vi "KM_String Array Select.vi"(10 "Selector array":bool[](array[boolean]), 11 "Full array":string[](array[string])) -> (3 "Array":string[](array[string]))   [LabVIEW 2015]
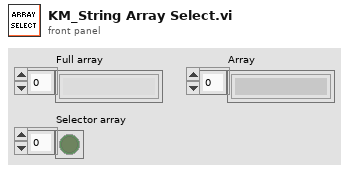
[diagram p1: front panel]
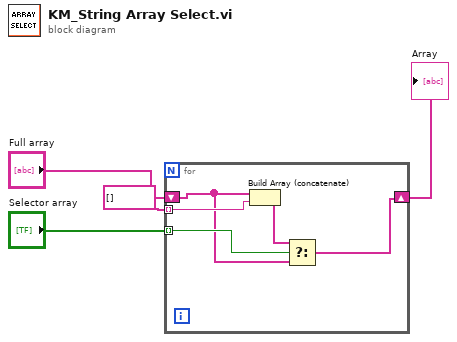
[diagram p0: block diagram]
diagram:
  n1 = for {
    tunnel: "Full array" -> [w8] mode=indexing
    tunnel: "Selector array" -> [w9] mode=indexing
    shift-right: [w5] -> w2
    shift-left: string[] [] -> [w6]
    n2 = Build Array (concatenate)(w6, w8) -> (w7:string[])
    n3 = Select(t=w7, s=w9, f=w6) -> (s? t:f=w5:string[])
  }
  "Array" <- w2
